vi "Read Loop Period (ms).vi"(11 "Application in":refnum<class "Application.lvclass">) -> (2 "Loop Period (ms)":u16=100 min=1 max=5000, 3 "Application out":refnum<class "Application.lvclass">)   [LabVIEW 2013, in "Application.lvlib" / "Application.lvclass"]
uses:
  <userlib>/Common/Component/Application/Application/Application.lvclass
  <userlib>/Common/Component/Application/Application/Application.lvclass/Application.ctl
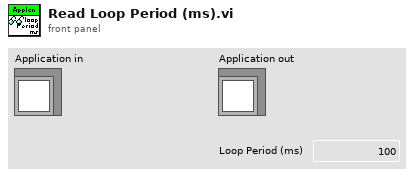
[diagram p1: front panel]
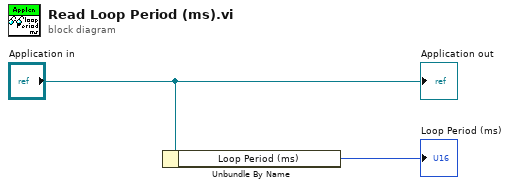
[diagram p0: block diagram]
diagram:
  n1 = Unbundle By Name("Application in") -> ("Loop Period (ms)"=→"Loop Period (ms)":u16)
  "Application out" <- "Application in"
